vi "Tag Engine Test 3.vi"() -> ()   [LabVIEW 2020]
doc: "_Test_"
uses:
  Tag/Tag.lvclass/Tag.ctl
  20c6578c-4bd2-4559-8eb7-19bb61ff37ef.vi
  04a4cf95-a8fd-4fdc-961e-714608aacd3b.vi
  9caf1127-d5a6-40b5-bb56-68120de02a46.vi
  87cc020f-e60a-492d-9f9a-d17fac712b41.vi
  a32eeae9-b076-4228-86a7-a13287abedbe.vi
  3ad88a87-eff0-441b-814b-2b02c807fa8e.vi
  544cd850-60c9-4755-8e92-da0a88e05141.vi
  882321c8-2844-4045-b5cd-05a057c0d04f.vi
  Tag/Construct.vi
  Core/Get Tag Value_ByRef.vi
  Tag/Read Value.vi
  Tag/Read Timestamp.vi
  Tag/Set Properties from Initial.vi
  Core/Add Tag.vi
  <vilib>/Utility/Data Type/Get Type Information.vi
  <vilib>/JDP Science/JSONtext/Variant to JSON Text.vi
  Tag/Tag.lvclass
  Core/Tag Core.lvclass
  Tag Engine.lvlib
panel:
  out "Value 5":variant
  out "Value 4":string
  out "Value 2":dbl[][][](array[numeric])
  out "Value 3":variant
  out "Value 2":string
  out "error out":errorcluster
  out "Value":cluster{"test1":i32, "test2":dbl}
  out "error out 2":errorcluster
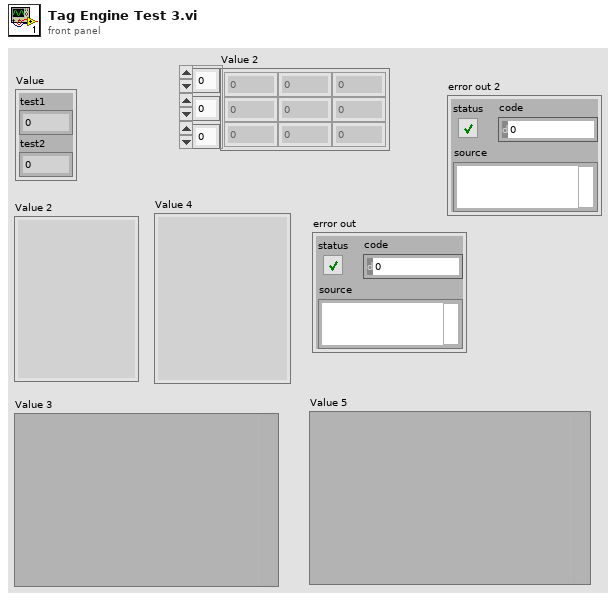
[diagram p1: front panel]
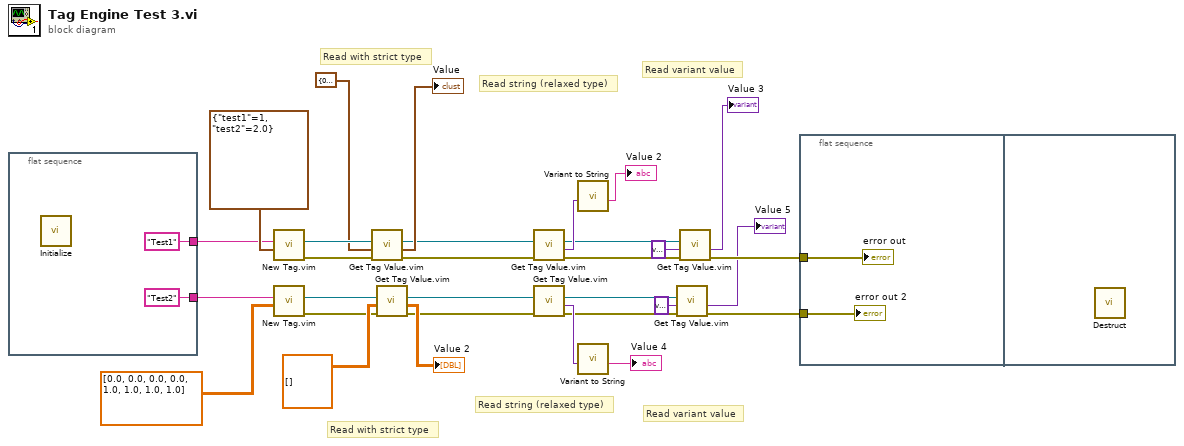
[diagram p0: block diagram]
diagram:
  # "Read variant value"
  # "Read with strict type"
  # "Read string (relaxed type)"
  # "Read variant value"
  # "Read string (relaxed type)"
  # "Read with strict type"
  n1 = flat-sequence {
    tunnel: ["Test1" ("Name")] -> w28
    tunnel: ["Test2" ("Name")] -> w27
    frame #0 {
      n2 = call "Initialize.vi"() -> ()  [unwired: 11 in, 1 out]
    }
  }
  n3 = call "New Tag.vim"("Initial Value"=cluster{"test1":i32, "test2":dbl} {"test1"=1, "test2"=2.0}, "Tag Name"=w28) -> ("error out"=w22:errorcluster, "Tag Ref out"=w24:refnum<data-value>)  [unwired: 8 in]
  n4 = call "New Tag.vim"("Initial Value"=dbl[][][] [[[0.0, 0.0], [0.0, 0.0]], [[1.0, 1.0], [1.0, 1.0]]], "Tag Name"=w27) -> ("error out"=w10:errorcluster, "Tag Ref out"=w12:refnum<data-value>)  [unwired: 8 in]
  n5 = call "Get Tag Value.vim"("error in (no error)"=w22, "Default (Void)"=cluster{"test1":i32, "test2":dbl} {"test1"=0, "test2"=0.0}, "Tag Name(s)/Ref(s)"=w24) -> ("error out"=w19:errorcluster, "Value(s)"=→"Value":cluster{"test1":i32, "test2":dbl}, "Tag Ref(s) out"=w20:refnum<data-value>)  [unwired: 5 in, 1 out]
  n6 = call "Get Tag Value.vim"("error in (no error)"=w10, "Default (Void)"=dbl[][][] [], "Tag Name(s)/Ref(s)"=w12) -> ("error out"=w7:errorcluster, "Value(s)"=→"Value 2":dbl[][][], "Tag Ref(s) out"=w8:refnum<data-value>)  [unwired: 5 in, 1 out]
  n7 = call "Get Tag Value.vim"("error in (no error)"=w19, "Tag Name(s)/Ref(s)"=w20) -> ("error out"=w17:errorcluster, "Value(s)"=w18:variant, "Tag Ref(s) out"=w15:refnum<data-value>)  [unwired: 6 in, 1 out]
  n8 = call "Get Tag Value.vim"("error in (no error)"=w7, "Tag Name(s)/Ref(s)"=w8) -> ("error out"=w5:errorcluster, "Value(s)"=w6:variant, "Tag Ref(s) out"=w4:refnum<data-value>)  [unwired: 6 in, 1 out]
  n9 = call "Variant to String.vi"("Variant Value"=w18) -> ("String Value"=→"Value 2":string)  [unwired: 9 in, 1 out]
  n10 = call "Variant to String.vi"("Variant Value"=w6) -> ("String Value"=→"Value 4":string)  [unwired: 9 in, 1 out]
  n11 = call "Get Tag Value.vim"("error in (no error)"=w5, "Default (Void)"=variant, "Tag Name(s)/Ref(s)"=w4) -> ("error out"=w1:errorcluster, "Value(s)"=→"Value 5":variant)  [unwired: 5 in, 2 out]
  n12 = call "Get Tag Value.vim"("error in (no error)"=w17, "Default (Void)"=variant, "Tag Name(s)/Ref(s)"=w15) -> ("error out"=w13:errorcluster, "Value(s)"=→"Value 3":variant)  [unwired: 5 in, 2 out]
  n13 = flat-sequence {
    tunnel: w1 -> [w34]
    tunnel: w13 -> [w33]
    frame #0 {
      "error out 2" <- w34
      "error out" <- w33
    }
    frame #1 {
      n14 = call "Destruct.vi"() -> ()  [unwired: 11 in, 1 out]
    }
  }
